vi "Tarea 7.vi"() -> ()   [LabVIEW 2019]
panel:
  out "Code String Out":string
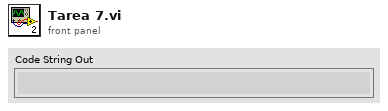
[diagram p1: front panel]
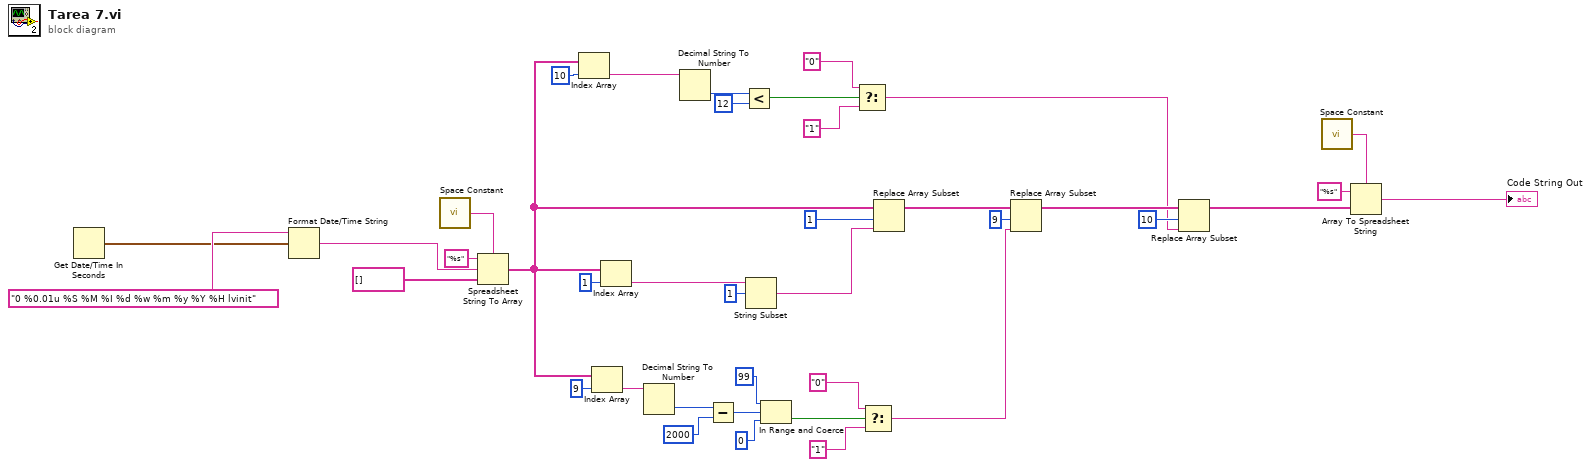
[diagram p0: block diagram]
diagram:
  n1 = Get Date/Time In Seconds() -> (seconds since 1Jan1904=w25:timestamp)
  n2 = Format Date/Time String(time format string (%c)="0 %0.01u %S %M %I %d %w %m %y %Y %H lvinit", seconds (now)=w25) -> (date/time string=w38:string)  [unwired: 1 in]
  n3 = call <vilib>:"Space Constant.vi"() -> ("String"=w27:string)
  n4 = Spreadsheet String To Array(delimiter (Tab)=w27, format string="%s", spreadsheet string=w38, array type (2D Dbl)=string[] []) -> (array=w10:string[])
  n5 = Index Array "Index Array"(array=w10, index=10) -> (element=w7:string)
  n6 = Index Array "Index Array"(array=w10, index=9) -> (element=w23:string)
  n7 = Index Array "Index Array"(array=w10, index=1) -> (element=w34:string)
  n8 = Decimal String To Number(string=w23) -> (number=w22:i32)  [unwired: 2 in, 1 out]
  n9 = Decimal String To Number(string=w7) -> (number=w6:i32)  [unwired: 2 in, 1 out]
  n10 = Subtract(x=w22, y=2000) -> (x-y=w20:i32)
  n11 = Less?(x=w6, y=12) -> (x < y?=w2:bool)
  n12 = String Subset(string=w34, offset (0)=1) -> (substring=w32:string)  [unwired: 1 in]
  n13 = In Range and Coerce(upper limit=99, x=w20, lower limit=0 ("x-y")) -> (In Range?=w17:bool)  [unwired: 1 out]
  n14 = Select(t="0", s=w2, f="1") -> (s? t:f=w1:string)
  n15 = Select(t="0", s=w17, f="1") -> (s? t:f=w12:string)
  n16 = Replace Array Subset "Replace Array Subset"(array=w10, new element=w32, index=1) -> (w30:string[])
  n17 = Replace Array Subset "Replace Array Subset"(array=w30, new element=w12, index=9) -> (w14:string[])
  n18 = Replace Array Subset "Replace Array Subset"(array=w14, new element=w1, index=10) -> (w9:string[])
  n19 = call <vilib>:"Space Constant.vi"() -> ("String"=w28:string)
  n20 = Array To Spreadsheet String(delimiter (Tab)=w28, array=w9, 3:"%s" ("format string")) -> (spreadsheet string=→"Code String Out":string)
